vi "Add Multiple Wheels to Steering Frame.vi"(5 "x positions":dbl[](array[numeric]), 6 "frame angles (rad)":dbl[](array[numeric]), 7 "y positions":dbl[](array[numeric]), 8 "error in (no error)":errorcluster, 10 "wheels":refnum<class "NI_Robotics_Wheel.lvclass">[](array[class]), 11 "steering frame in":refnum<class "NI_Robotics_Steering Frame.lvclass">) -> (0 "error out":errorcluster, 3 "steering frame out":refnum<class "NI_Robotics_Steering Frame.lvclass">)   [LabVIEW 2017, in "NI_Robotics_Steering Frame.lvclass"]
doc: "Adds the wheel or wheels you specify to <B>steering frame in</B>. You must manually select the polymorphic instance to use."
uses:
  <vilib>/robotics/Steering/Steering Frame/NI_Robotics_Steering Frame.lvclass
  <vilib>/robotics/Steering/Wheel/NI_Robotics_Wheel.lvclass
  <vilib>/robotics/Steering/Steering Frame/Wheel Orientation.ctl
  <vilib>/robotics/Steering/Wheel/Wheel State.ctl
  <vilib>/robotics/Steering/Wheel/NI_Robotics_Wheel.lvclass/NI_Robotics_Wheel.ctl
  <vilib>/robotics/Steering/Steering Frame/NI_Robotics_Steering Frame.lvclass/NI_Robotics_Steering Frame.ctl
  <vilib>/Analysis/coordinate.llb/Wrap Angle (scalar).vi
  <vilib>/robotics/Utilities/NI_Robotics Utilities.lvlib
  <vilib>/Analysis/NI_AAL_Angle.lvlib
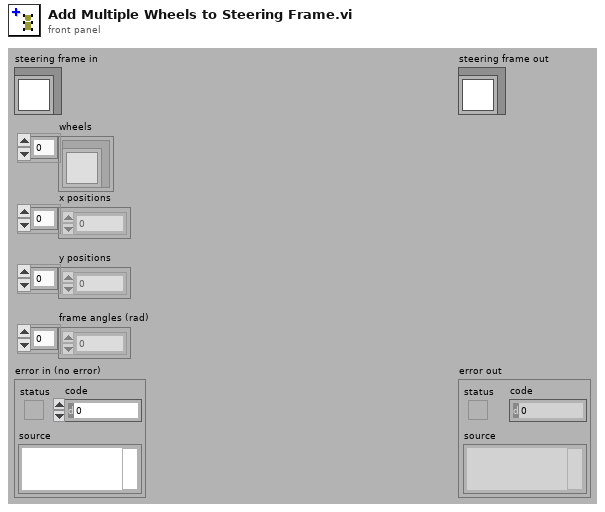
[diagram p1: front panel]
types:
  T1 = typedef "NI_Robotics_Wheel.lvclass/Wheel State.ctl" = cluster{"wheel name":string, "forward angular velocity":dbl, "caster angular velocity":dbl, "caster wheel angle (rad)":dbl, "steering angle (rad)":dbl}
  T2 = typedef "NI_Robotics_Steering Frame.lvclass/Wheel Orientation.ctl" = cluster{"wheel":refnum<class "NI_Robotics_Wheel.lvclass">, "x position":dbl, "y position":dbl, "frame angle (rad)":dbl}
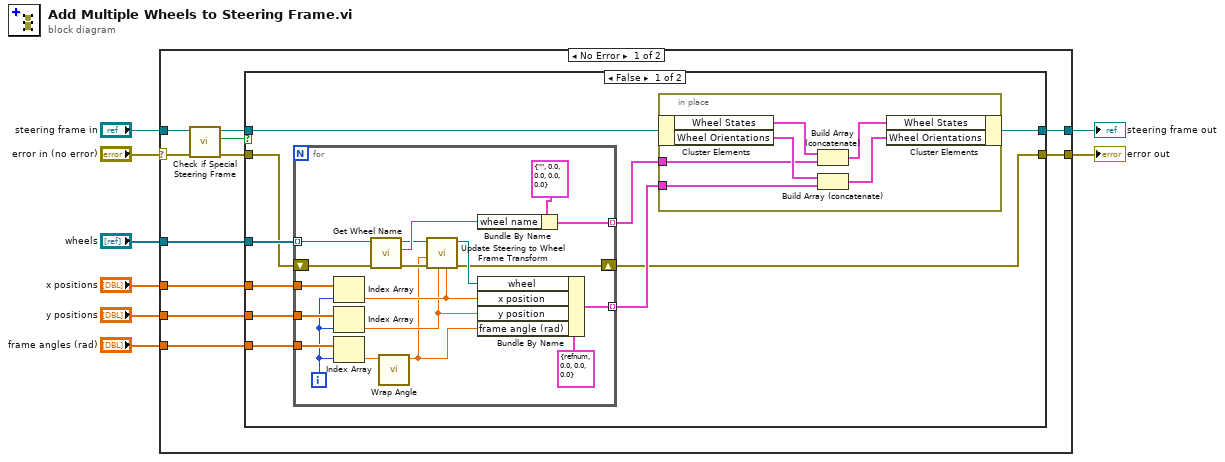
[diagram p0: block diagram]
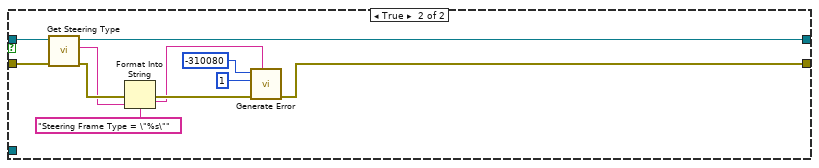
[diagram p2: hidden frame]
diagram:
  n1 = case shown="No Error" "error in (no error)" {
    selector: "error in (no error)" -> [w16 w67]
    tunnel: [w13 w67] -> w7
    tunnel: [w19 w66] -> w5
    tunnel: "steering frame in" -> [w18 w66]
    tunnel: "wheels" -> [w12 _]
    tunnel: "x positions" -> [w11 _]
    tunnel: "y positions" -> [w10 _]
    tunnel: "frame angles (rad)" -> [w9 _]
    frame No Error {
      n2 = call-dynamic "Check if Special Steering Frame.vi"("error in (no error)"=w16, "steering frame in"=w18) -> ("error out"=w14:errorcluster, "special?"=w15:bool, "steering frame out"=w17:refnum<class "NI_Robotics_Steering Frame.lvclass">)  [unwired: 7 in]
      n3 = case shown="False" w15 {
        tunnel: [w21 w58] -> w19
        tunnel: w17 -> [w29 w59]
        tunnel: w14 -> [w24 w57]
        tunnel: [w23 w65] -> w13
        tunnel: w12 -> [w26 _]
        tunnel: w11 -> [w28 _]
        tunnel: w10 -> [w27 _]
        tunnel: w9 -> [w20 _]
        frame False {
          n4 = for {
            tunnel: w26 -> [w46] mode=indexing
            tunnel: w28 -> [w37]
            tunnel: w27 -> [w35]
            tunnel: w20 -> [w33]
            tunnel: [w47] -> w25 mode=indexing
            shift-right: [w38] -> w23
            shift-left: w24 -> [w45]
            tunnel: [w42] -> w22 mode=indexing
            i -> [w32]
            n5 = Index Array(array=w37, index=w32) -> (element=w36:dbl)
            n6 = Index Array(array=w35, index=w32) -> (element=w34:dbl)
            n7 = Index Array(array=w33, index=w32) -> (element=w31:dbl)
            n8 = call <vilib>:"Get Wheel Name.vi"("error in (no error)"=w45, "wheel in"=w46) -> ("error out"=w39:errorcluster, "wheel name"=w43:string, "wheel out"=w41:refnum<class "NI_Robotics_Wheel.lvclass">)  [unwired: 7 in]
            n9 = call-poly <vilib>:"Wrap Angle.vi"("angle in"=w31) -> ("angle out"=w30:dbl)  [unwired: 9 in, 1 out]
            n10 = call <vilib>:"Update Steering to Wheel Frame Transform.vi"("x wheel position"=w36, "y wheel position"=w34, "error in (no error)"=w39, "wheel frame angle (rad)"=w30, "wheel in"=w41) -> ("error out"=w38:errorcluster, "wheel out"=w40:refnum<class "NI_Robotics_Wheel.lvclass">)  [unwired: 5 in]
            n11 = Bundle By Name(cluster=T1 {"wheel name"="", "forward angular velocity"=0.0, "caster angular velocity"=0.0, "caster wheel angle (rad)"=0.0, "steering angle (rad)"=0.0} ("wheel state"), "wheel name"=w43) -> (w42:T1)
            n12 = Bundle By Name(cluster=T2 {"wheel"=refnum, "x position"=0.0, "y position"=0.0, "frame angle (rad)"=0.0} ("wheel orientation"), "wheel"=w40, "x position"=w36, "y position"=w34, "frame angle (rad)"=w30) -> (w47:T2)
          }
          n13 = in-place {
            in-place-border: w25 -> [w53]
            in-place-border: w22 -> [w49]
            n14 = in-place-cluster #1(w29) -> ("Wheel States"=w51:T1[], "Wheel Orientations"=w54:T2[])
            n15 = Build Array (concatenate)(w51, w49) -> (w50:T1[])
            n16 = Build Array (concatenate)(w54, w53) -> (w52:T2[])
            n17 = in-place-cluster #1("Wheel States"=w50, "Wheel Orientations"=w52) -> (w21:refnum<class "NI_Robotics_Steering Frame.lvclass">)
          }
        }
        frame True {
          n18 = call-dynamic "Get Steering Type.vi"("error in (no error)"=w57, "steering frame in"=w59) -> ("error out"=w62:errorcluster, "steering type"=w61:string, "steering frame out"=w58:refnum<class "NI_Robotics_Steering Frame.lvclass">)  [unwired: 7 in]
          n19 = Format Into String(format string="Steering Frame Type = \"%s\"", error in=w62, w61) -> (resulting string=w55:string, error out=w56:errorcluster)  [unwired: 1 in]
          n20 = call <vilib>:"Generate Error.vi"("<append> (\"\")"=w55, "error in (no error)"=w56, "chain levels to remove (1)"=1, "code"=-310080) -> ("error out"=w65:errorcluster)  [unwired: 7 in]
        }
      }
    }
    frame Error {
    }
  }
  "error out" <- w7
  "steering frame out" <- w5
